vi "DAC Configure.vi"(8 "error in":errorcluster, 11 "DAC HTS dU in":refnum<class "DAC HTS dU.lvclass">) -> (0 "error out":errorcluster, 3 "DAC HTS dU out":refnum<class "DAC HTS dU.lvclass">)   [LabVIEW 2019, in "DAC.lvlib" / "DAC HTS dU.lvclass"]
uses:
  DAC HTS dU.lvclass
  C:/Users/krio/Documents/LV_Projects/test-stand/App/DAC/DAC.lvclass
  DAC.lvclass/DAC.ctl
  DAC HTS dU.lvclass/DAC HTS dU.ctl
  <vilib>/Instr/_visa.llb/VISA Configure Serial Port (Instr).vi
  DAC.lvclass
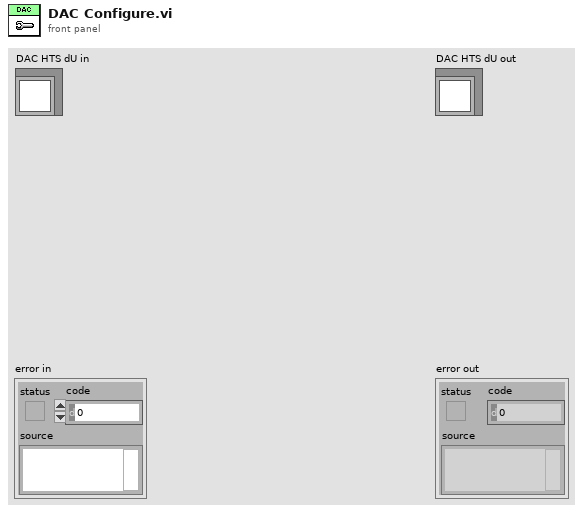
[diagram p1: front panel]
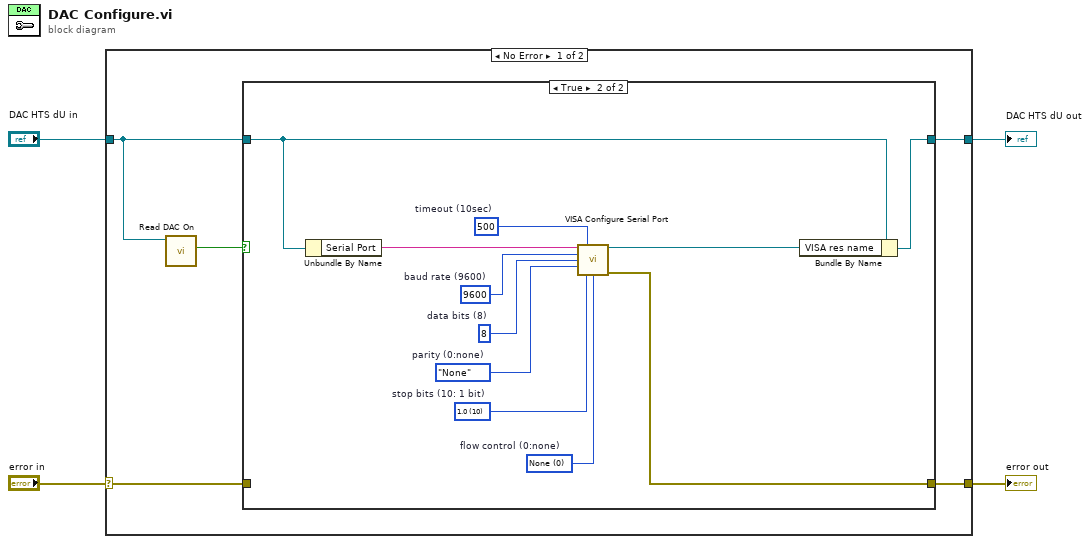
[diagram p0: block diagram]
diagram:
  n1 = case shown="No Error" "error in" {
    selector: "error in" -> [w6 w24]
    tunnel: [w5 w24] -> w4
    tunnel: [w7 w23] -> w3
    tunnel: "DAC HTS dU in" -> [w9 w23]
    frame No Error {
      n2 = call "Read DAC On.vi"("DAC in"=w9) -> ("DAC On"=w8:bool)  [unwired: 8 in, 2 out]
      n3 = case shown="True" w8 {
        tunnel: w9 -> [w11 w22]
        tunnel: [w11 w21] -> w7
        tunnel: w6 -> [w10 _]
        tunnel: [w10 w14] -> w5
        frame False {
          # "Temperature measurement is off."
        }
        frame True {
          w12 = u16 0 items=["None", "XON/XOFF", "RTS/CTS", "XON/XOFF & RTS/CTS", "DTR/DSR", "XON/XOFF & DTR/DSR"]  # flow control (0:none)
          w13 = u32 500  # timeout (10sec)
          w17 = u16 10 items=["1.0"=10, "1.5"=15, "2.0"=20]  # stop bits (10: 1 bit)
          w18 = enum16{"None", "Odd", "Even", "Mark", "Space"}."None"  # parity (0:none)
          w19 = u16 8  # data bits (8)
          w20 = u32 9600  # baud rate (9600)
          # "Temperature measurement is on."
          n4 = Unbundle By Name(w22) -> ("Serial Port"=w16:string)
          n5 = call-poly "VISA Configure Serial Port"("VISA resource name"=w16, "timeout (10sec)"=w13, "baud rate (9600)"=w20, "data bits (8)"=w19, "parity (0:none)"=w18, "stop bits (10: 1 bit)"=w17, "flow control (0:none)"=w12) -> ("VISA resource name out"=w15:refnum<visa-resource-name>, "error out"=w14:errorcluster)  [unwired: 7 in]
          n6 = Bundle By Name(cluster=w22, "VISA res name"=w15) -> (w21:refnum<class "DAC HTS dU.lvclass">)
        }
      }
    }
    frame Error {
    }
  }
  "error out" <- w4
  "DAC HTS dU out" <- w3
